vi "PS Notifier.vi"(2 "Status":cluster{bool, bool, "Ramp Status":u16, bool}, 3 "Field [T]":dbl caption="Current [kA]" format="%.5f") -> ()   [LabVIEW 2020]
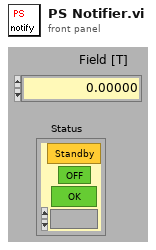
[diagram p1: front panel]
types:
  T1 = cluster{"Field [T]":dbl, "Status":cluster{bool, bool, "Ramp Status":u16, bool}}
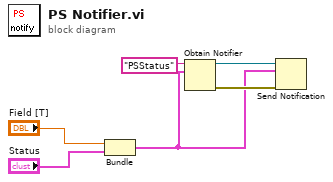
[diagram p0: block diagram]
diagram:
  n1 = Bundle("Field [T]"="Field [T]", "Status"="Status") -> (w1:T1)  [unwired: 1 in]
  n2 = Obtain Notifier(name (unnamed)="PSStatus", notification data type=w1) -> (notifier out=w3:refnum<notifier>, error out=w2:errorcluster)  [unwired: 2 in, 1 out]
  n3 = Send Notification(notification=w1, notifier=w3, error in (no error)=w2) -> ()  [unwired: 2 out]
